vi "From table array.vi"(0 "Table Array in":string[][](array[string])) -> (1 "Names":string[](array[string]), 2 "Costs":dbl[][](array[numeric]), 3 "Days":bool[][](array[boolean]))   [LabVIEW 2015]
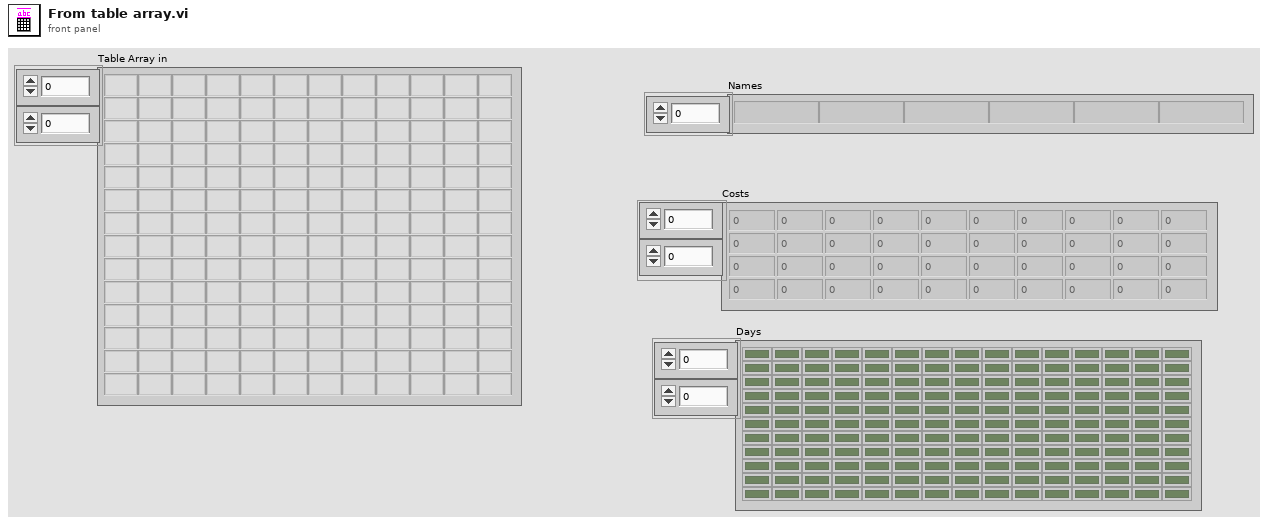
[diagram p1: front panel]
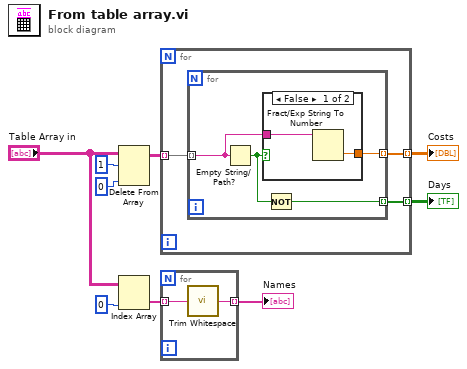
[diagram p0: block diagram]
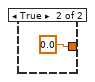
[diagram p2: hidden frame]
diagram:
  n1 = Delete From Array(array="Table Array in", length=1, index (col)=0 ("disabled index (col)")) -> (array with subset deleted=w7:string[][])  [unwired: 1 in, 1 out]
  n2 = Index Array(array="Table Array in", index (col)=0 ("disabled index (col)")) -> (element=w2:string[])  [unwired: 1 in]
  n3 = for {
    tunnel: w7 -> [w12] mode=indexing
    tunnel: [w11] -> w8 mode=indexing
    tunnel: [w10] -> w9 mode=indexing
    n4 = for {
      tunnel: w12 -> [w16] mode=indexing
      tunnel: [w15] -> w11 mode=indexing
      tunnel: [w13] -> w10 mode=indexing
      n5 = Empty String/Path?(string/path=w16) -> (empty?=w14:bool)
      n6 = case shown="False" w14 {
        tunnel: w16 -> [w18 _]
        tunnel: [w17 0.0] -> w15
        frame False {
          n7 = Fract/Exp String To Number(string=w18) -> (number=w17:dbl)  [unwired: 3 in, 1 out]
        }
        frame True {
        }
      }
      n8 = Not(x=w14) -> (.not. x?=w13:bool)
    }
  }
  "Days" <- w9
  "Costs" <- w8
  n9 = for {
    tunnel: w2 -> [w21] mode=indexing
    tunnel: [w20] -> w1 mode=indexing
    n10 = call <vilib>:"Trim Whitespace.vi"("string"=w21) -> ("trimmed string"=w20:string)  [unwired: 1 in]
  }
  "Names" <- w1
